vi "picomotor_driver.vi"() -> ()   [LabVIEW 2014]
uses:
  C:/Program Files/Newport/Piezo Motion Control/Newport AG-UC2-UC8 Applet/Samples/LabVIEW 2009/AgilisCmdLib.dll
  Program Files/Newport/Piezo Motion Control/Newport AG-UC2-UC8 Applet/Samples/LabVIEW 2009/AgilisCmdLib.dll
panel:
  out "Doing step move?":bool
  out "Jogging?":bool
  in  "Number of smaller steps":i32
  in  "Channel:":bool
  in  "Direction":bool
  in  "Stop Contoller?":bool
  in  "Start Jog":bool
  in  "Jog Step Amplitude (0-50)":i32 min=0 max=50 step=1
  in  "Jog Mode":T1(ring)
  in  "Control Rate (ms)":u32=20
  in  "Delay Time (s)":dbl=1.0
  in  "Small step size":i64
  in  "Stop steps?":bool
  in  "Do Steps?":bool
  in  "Stop Jog":bool
  out "STATUS":string
  out "ControllerVersion":string="AG-UC2 v2.2.0"
  in  "Instrument Key":string="COM9"
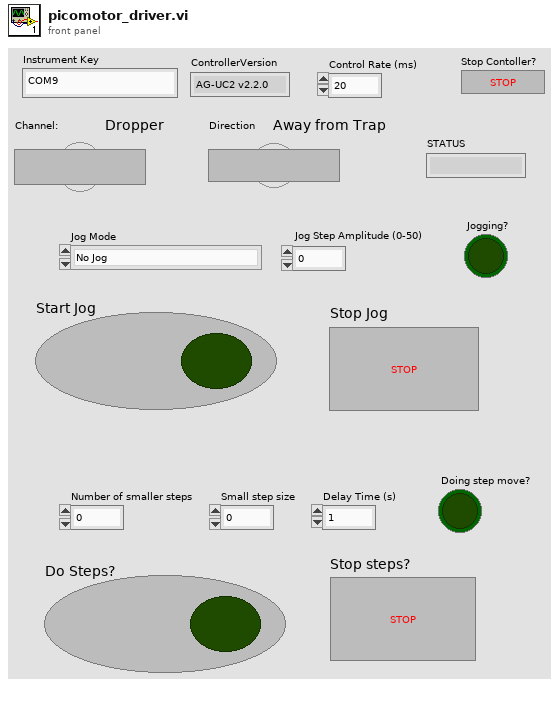
[diagram p1: front panel]
types:
  T1 = enum16{"No Jog", "5 steps/s at defined amp", "100 steps/s at max amp", "1700 steps/s at max amp", "666 steps/s at defined amp"}
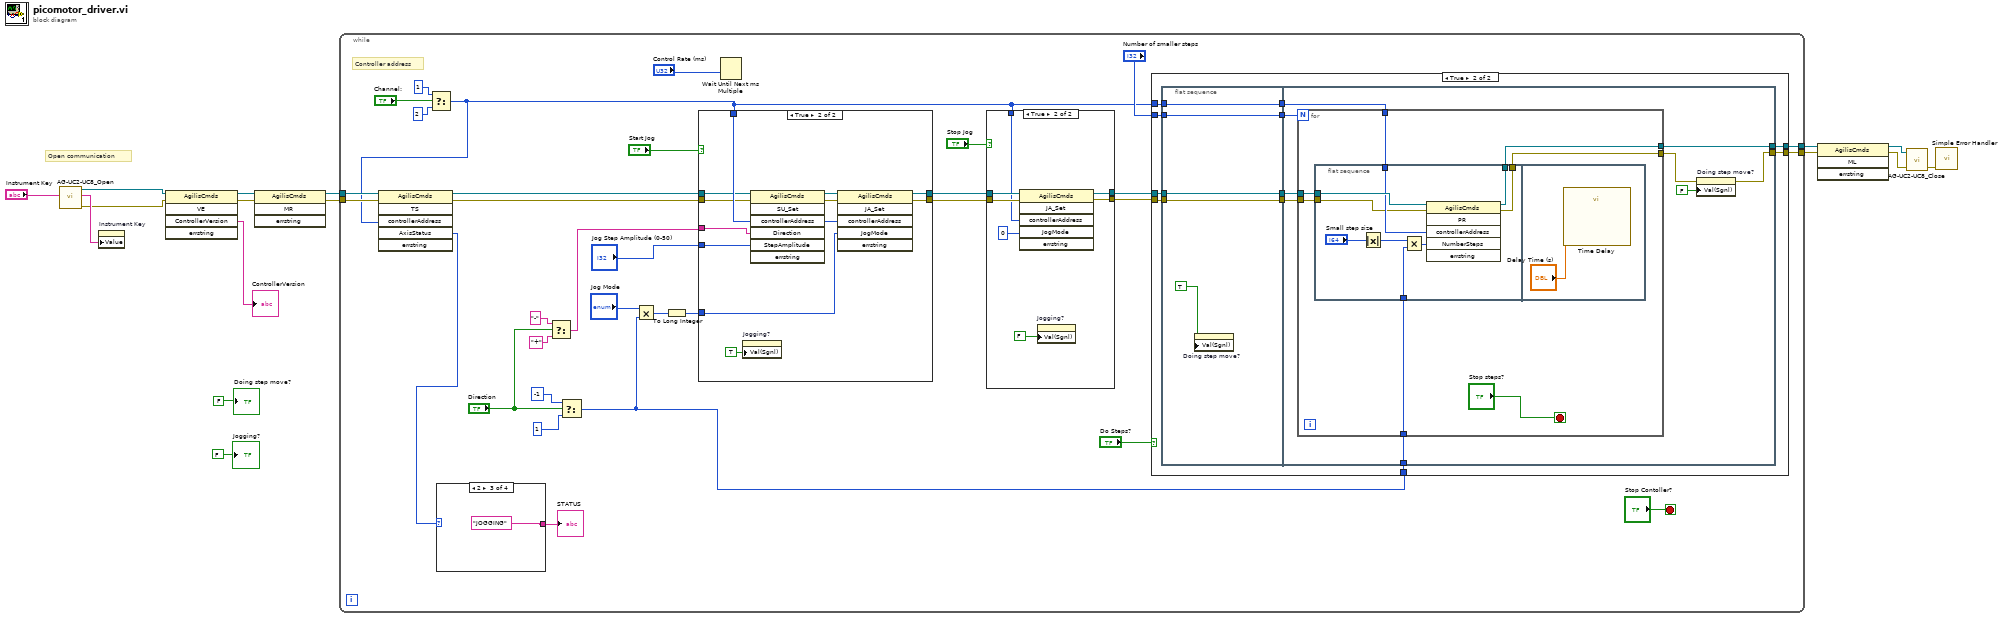
[diagram p0: block diagram]
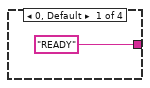
[diagram p2: hidden frame]
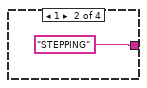
[diagram p3: hidden frame]
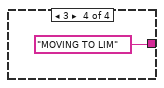
[diagram p4: hidden frame]
diagram:
  # "Open communication"
  n1 = call "AG-UC2-UC8_Open.vi"("Instrument Key IN"="Instrument Key") -> ("error out"=w14:errorcluster, "Instrument Key OUT"=w15:string, "AG-UC2-UC8 Reference"=w13:refnum<k24>)  [unwired: 3 in, 1 out]
  n2 = property on="Instrument Key" class="Str"("Value"=w15) -> ()  [unwired: 2 in, 2 out]
  n3 = invoke class="AgilisCmds" method="VE"(reference=w13, error in=w14) -> (reference out=w8:refnum<k24>, error out=w7:errorcluster, "ControllerVersion"=→"ControllerVersion":string)  [unwired: 3 in, 2 out]
  n4 = invoke class="AgilisCmds" method="MR"(reference=w8, error in=w7) -> (reference out=w6:refnum<k24>, error out=w5:errorcluster)  [unwired: 2 in, 2 out]
  n5 = while {
    tunnel: w6 -> [w23]
    tunnel: w5 -> [w22]
    tunnel: [w30] -> w4
    tunnel: [w29] -> w3
    stop <- "Stop Contoller?" stop-if-true
    # "Controller address"
    n6 = Select(t=1, s="Channel:", f=2) -> (s? t:f=w21:i32)
    n7 = invoke class="AgilisCmds" method="TS"(reference=w23, error in=w22, "controllerAddress"=w21) -> (reference out=w20:refnum<k24>, error out=w19:errorcluster, "AxisStatus"=w18:i32)  [unwired: 3 in, 3 out]
    n8 = case shown="2" w18 {
      tunnel: ["READY" "STEPPING" "JOGGING" "MOVING TO LIM"] -> w17
      frame 0, Default {
      }
      frame 1 {
      }
      frame 2 {
      }
      frame 3 {
      }
    }
    "STATUS" <- w17
    n9 = Select(t="-", s="Direction", f="+") -> (s? t:f=w35:string)
    n10 = Select(t=i64 -1, s="Direction", f=i64 1) -> (s? t:f=w39:i64)
    n11 = Multiply(x="Jog Mode", y=w39) -> (x*y=w31:i64)
    n12 = To Long Integer(number=w31) -> (32bit integer=w32:i32)
    n13 = case shown="True" "Start Jog" {
      tunnel: "Jog Step Amplitude (0-50)" -> [_ w119]
      tunnel: w32 -> [_ w118]
      tunnel: w21 -> [_ w117]
      tunnel: w20 -> [w108 w116]
      tunnel: w19 -> [w107 w115]
      tunnel: [w108 w113] -> w28
      tunnel: [w107 w112] -> w27
      tunnel: w35 -> [_ w114]
      frame False {
      }
      frame True {
        n14 = property on="Jogging?" class="Bool (strict)"("Val(Sgnl)"=TRUE ("Value (Signaling)")) -> ()  [unwired: 2 in, 2 out]
        n15 = invoke class="AgilisCmds" method="SU_Set"(reference=w116, error in=w115, "controllerAddress"=w117, "Direction"=w114, "StepAmplitude"=w119) -> (reference out=w110:refnum<k24>, error out=w111:errorcluster)  [unwired: 2 in, 5 out]
        n16 = invoke class="AgilisCmds" method="JA_Set"(reference=w110, error in=w111, "controllerAddress"=w117, "JogMode"=w118) -> (reference out=w113:refnum<k24>, error out=w112:errorcluster)  [unwired: 2 in, 4 out]
      }
    }
    n17 = Wait Until Next ms Multiple(millisecond multiple="Control Rate (ms)") -> ()  [unwired: 1 out]
    n18 = case shown="True" "Stop Jog" {
      tunnel: w28 -> [w55 w62]
      tunnel: w27 -> [w54 w61]
      tunnel: [w55 w60] -> w25
      tunnel: [w54 w59] -> w24
      tunnel: w21 -> [_ w57]
      frame False {
      }
      frame True {
        n19 = invoke class="AgilisCmds" method="JA_Set"(reference=w62, error in=w61, "controllerAddress"=w57, "JogMode"=0) -> (reference out=w60:refnum<k24>, error out=w59:errorcluster)  [unwired: 2 in, 4 out]
        n20 = property on="Jogging?" class="Bool (strict)"("Val(Sgnl)"=FALSE ("Value (Signaling)")) -> ()  [unwired: 2 in, 2 out]
      }
    }
    n21 = case shown="True" "Do Steps?" {
      tunnel: "Number of smaller steps" -> [_ w71]
      tunnel: [w64 w70] -> w30
      tunnel: [w63 w69] -> w29
      tunnel: w39 -> [_ w68]
      tunnel: w21 -> [_ w67]
      tunnel: w25 -> [w64 w66]
      tunnel: w24 -> [w63 w65]
      frame False {
      }
      frame True {
        n22 = flat-sequence {
          tunnel: w67 -> [w78]
          tunnel: w66 -> [w79]
          tunnel: w71 -> [w80]
          tunnel: [w80] -> w75
          tunnel: [w79] -> w74
          tunnel: [w78] -> w73
          tunnel: w65 -> [w76]
          tunnel: [w76] -> w72
          tunnel: [w81] -> w69
          tunnel: [w89] -> w70
          tunnel: w72 -> [w84]
          tunnel: w68 -> [w85]
          tunnel: w73 -> [w86]
          tunnel: w74 -> [w87]
          tunnel: w75 -> [w88]
          frame #0 {
            n23 = property on="Doing step move?" class="Bool (strict)"("Val(Sgnl)"=TRUE ("Value (Signaling)")) -> ()  [unwired: 2 in, 2 out]
          }
          frame #1 {
            n24 = for {
              N: w88 -> [_]
              tunnel: w87 -> [w96]
              tunnel: w86 -> [w95]
              tunnel: [w94] -> w89
              tunnel: [w93] -> w82
              tunnel: w85 -> [w91]
              tunnel: w84 -> [w90]
              stop <- "Stop steps?" stop-if-true
              n25 = flat-sequence {
                tunnel: w96 -> [w105]
                tunnel: w95 -> [w104]
                tunnel: [w103] -> w94
                tunnel: [w102] -> w93
                tunnel: w91 -> [w100]
                tunnel: w90 -> [w97]
                frame #0 {
                  n26 = Absolute Value(x="Small step size") -> (abs(x)=w99:i64)
                  n27 = Multiply(x=w99, y=w100) -> (x*y=w101:i64)
                  n28 = invoke class="AgilisCmds" method="PR"(reference=w105, error in=w97, "controllerAddress"=w104, "NumberSteps"=w101) -> (reference out=w103:refnum<k24>, error out=w102:errorcluster)  [unwired: 2 in, 4 out]
                }
                frame #1 {
                  n29 = call "Time Delay"("Delay Time (s)"="Delay Time (s)") -> ()  [unwired: 10 in, 1 out]
                }
              }
            }
            n30 = property on="Doing step move?" class="Bool (strict)"(error in=w82, "Val(Sgnl)"=FALSE ("Value (Signaling)")) -> (error out=w81:errorcluster)  [unwired: 1 in, 1 out]
          }
        }
      }
    }
  }
  n31 = invoke class="AgilisCmds" method="ML"(reference=w4, error in=w3) -> (reference out=w11:refnum<k24>, error out=w10:errorcluster)  [unwired: 2 in, 2 out]
  n32 = call "AG-UC2-UC8_Close.vi"("error in (no error)"=w10, "AG-UC2-UC8 Reference"=w11) -> ("Error out"=w9:errorcluster)  [unwired: 2 in, 1 out]
  n33 = call <vilib>:"Simple Error Handler.vi"("error in (no error)"=w9) -> ()  [unwired: 4 in, 5 out]
  "Jogging?" <- FALSE ("Boolean")
  "Doing step move?" <- FALSE ("Boolean")
